vi "ProdaNG.Extract.U8[].vi"(0 "unsigned byte array":u8[](array[numeric]), 1 "Sizes":i32[](array[numeric])) -> (2 "Elements":string[](array[string]))   [LabVIEW 2016]
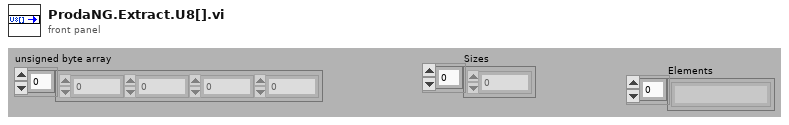
[diagram p1: front panel]
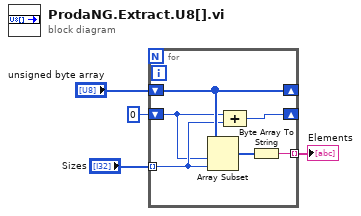
[diagram p0: block diagram]
diagram:
  n1 = for {
    shift-right: [w10] -> _
    shift-left: "unsigned byte array" -> [w10]
    tunnel: "Sizes" -> [w9] mode=indexing
    shift-right: [w8] -> _
    shift-left: 0 -> [w7]
    tunnel: [w5] -> w1 mode=indexing
    n2 = Array Subset(array=w10, index=w7, length=w9) -> (w6:u8[])
    n3 = Compound Arithmetic op=ADD(w7, w9) -> (w8:i32)
    n4 = Byte Array To String(unsigned byte array=w6) -> (string=w5:string)
  }
  "Elements" <- w1
